vi "Position Inspection Height slider.vi"(8 "error in (no error)":errorcluster, 10 "Circumnavigate ref":refnum<vi>, 11 "Slide Refnum":refnum<vi>) -> (0 "error out":errorcluster)   [LabVIEW 2014]
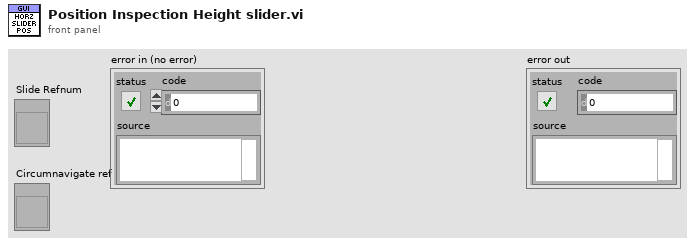
[diagram p1: front panel]
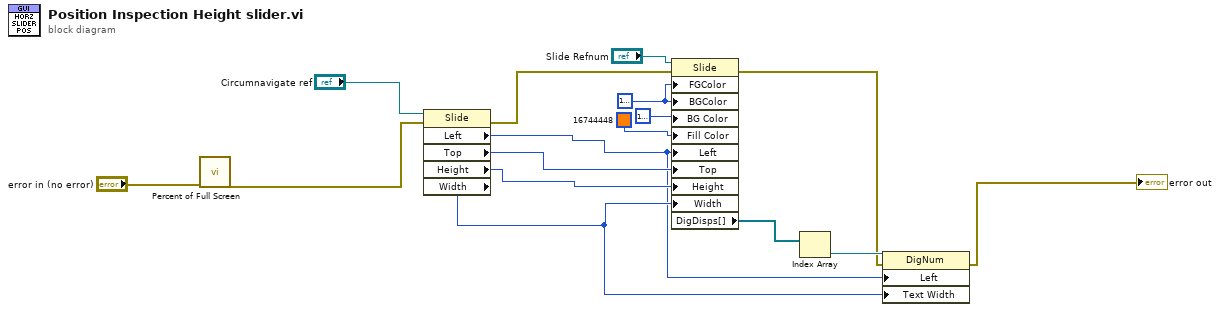
[diagram p0: block diagram]
diagram:
  w11 = u32 16777226
  n1 = call "Percent of Full Screen.vi"("error in (no error)"="error in (no error)") -> ("error out"=w3:errorcluster)  [unwired: 8 in, 2 out]
  n2 = property class="Slide"(reference="Circumnavigate ref", error in=w3) -> (error out=w14:errorcluster, "Left"=w1:i32, "Top"=w5:i32, "Height"=w2:u32, "Width"=w4:u32)  [unwired: 1 out]
  n3 = property class="Slide"(reference="Slide Refnum", error in=w14, "FGColor"=w11, "BGColor"=w11, "BG Color"=u32 16777228, "Fill Color"=u32 16744448, "Left"=w1, "Top"=w5, "Height"=w2, "Width"=w4) -> (error out=w7:errorcluster, "DigDisps[]"=w9:refnum<vi>[])  [unwired: 1 out]
  n4 = Index Array(array=w9) -> (element=w8:refnum<vi>)  [unwired: 1 in]
  n5 = property class="DigNum"(reference=w8, error in=w7, "Left"=w1, "Text Width"=w4) -> (error out=→"error out":errorcluster)  [unwired: 1 out]
